vi "MKS_PDR2000_write_read.vi"(0 "PDR2000 COM port":refnum<visa-resource-name>, 2 "Write string":string, 11 "error in (no error)":errorcluster) -> (4 "PDR2000 COM port out":refnum<visa-resource-name>, 13 "Read String":string, 15 "error out":errorcluster)   [LabVIEW 2019]
uses:
  <vilib>/regexp/Match Regular Expression.xnode
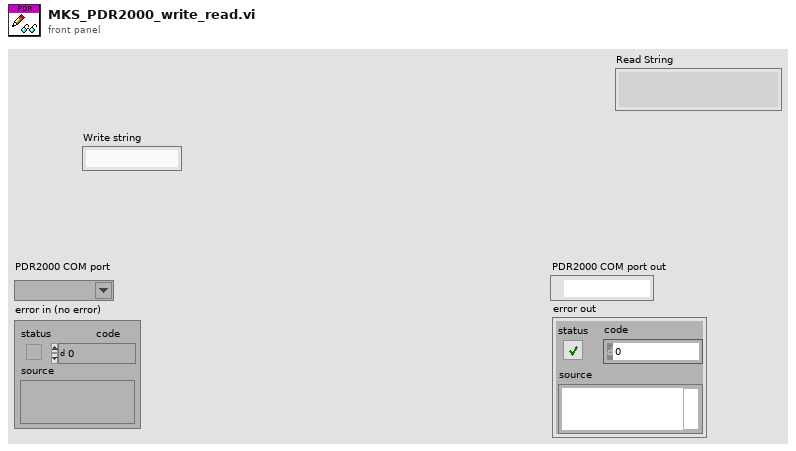
[diagram p1: front panel]
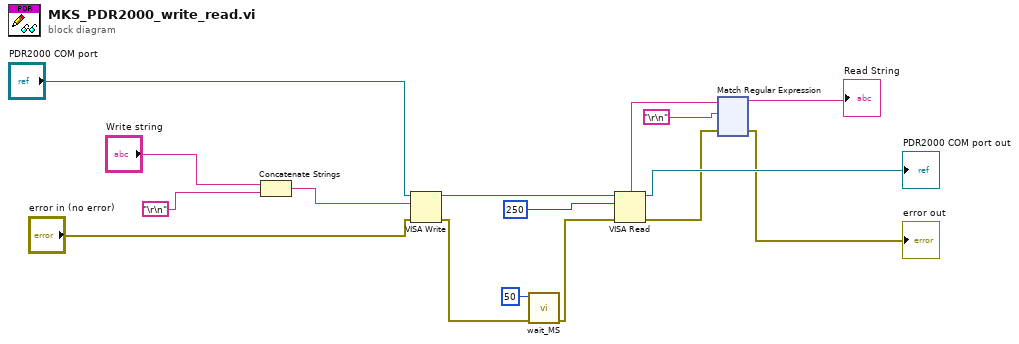
[diagram p0: block diagram]
diagram:
  n1 = Concatenate Strings("Write string", "\r\n") -> (w13:string)
  n2 = VISA Write(VISA resource name="PDR2000 COM port", write buffer=w13, error in (no error)="error in (no error)") -> (VISA resource name out=w10:refnum<visa-resource-name>, error out=w12:errorcluster)  [unwired: 1 out]
  n3 = call "wait_MS.vi"("error in (no error)"=w12, "milliseconds to wait"=u32 50) -> ("error out"=w11:errorcluster)  [unwired: 9 in]
  n4 = VISA Read(VISA resource name=w10, byte count=u32 250, error in (no error)=w11) -> (VISA resource name out=→"PDR2000 COM port out":refnum<visa-resource-name>, read buffer=w6:string, error out=w4:errorcluster)  [unwired: 1 out]
  n5 = xnode "Match Regular Expression"("input string"=w6, "regular expression"="\r\n", "error in"=w4) -> ("before match"=→"Read String":string, "error out"=→"error out":errorcluster)  [unwired: 3 in, 3 out]
